vi "Torque_FGV.vi"(9 "Selector FGV":enum16{"Leer", "Escribir"}(ring), 10 "Torque In":dbl) -> (2 "Torque Out":dbl)   [LabVIEW 2020]
panel:
  out "Torque In  2":dbl
  out "Torque In  2":dbl
  out "Torque In  2":dbl
  out "Torque In  2":dbl
  out "Torque In  2":dbl
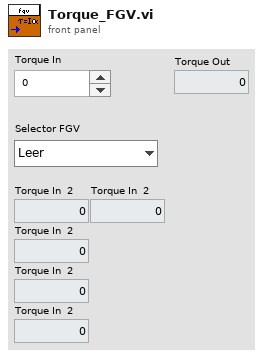
[diagram p1: front panel]
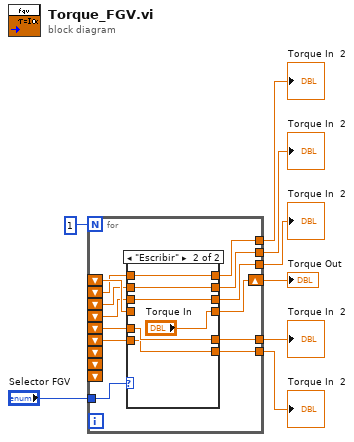
[diagram p0: block diagram]
diagram:
  n1 = for {
    N: 1 -> [_]
    shift-right: [w20] -> w6
    shift-left: _ -> [w19]
    tunnel: "Selector FGV" -> [w21]
    shift-left: _ -> [w18]
    shift-left: _ -> [w17]
    shift-left: _ -> [w16]
    shift-left: _ -> [w15]
    shift-left: _ -> [w14]
    shift-left: _ -> [_]
    shift-left: _ -> [_]
    shift-left: _ -> [_]
    tunnel: [w13] -> w5
    tunnel: [w12] -> w1
    tunnel: [w11] -> w2
    tunnel: [w10] -> w3
    tunnel: [w9] -> w4
    n2 = case shown="\"Escribir\"" w21 {
      tunnel: [w27 "Torque In"] -> w20
      tunnel: w19 -> [w27 _]
      tunnel: [w26 w32] -> w13
      tunnel: w18 -> [w26 w32]
      tunnel: [w25 w31] -> w12
      tunnel: w17 -> [w25 w31]
      tunnel: [w24 w30] -> w11
      tunnel: w16 -> [w24 w30]
      tunnel: [w23 w29] -> w10
      tunnel: w15 -> [w23 w29]
      tunnel: [w22 w28] -> w9
      tunnel: w14 -> [w22 w28]
      frame "Leer", Default {
      }
      frame "Escribir" {
      }
    }
  }
  "Torque Out" <- w6
  "Torque In  2" <- w5
  "Torque In  2" <- w4
  "Torque In  2" <- w3
  "Torque In  2" <- w2
  "Torque In  2" <- w1
